vi "Delete.vi"(0 "image in":refnum<class "MSC Image.lvclass">, 5 "error in (no error)":errorcluster) -> (19 "error out":errorcluster)   [LabVIEW 2014, in "MSC Image.lvclass"]
doc: "Closes the image reference and frees occupied memory.\nUse this function for each initialized image to prevent memory leaks."
uses:
  MSC Image.lvclass
  MSC Image.lvclass/MSC Image.ctl
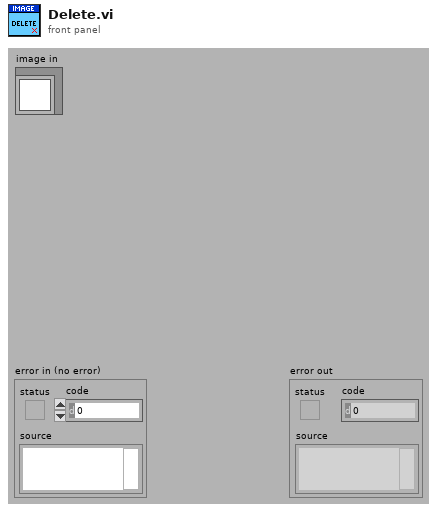
[diagram p1: front panel]
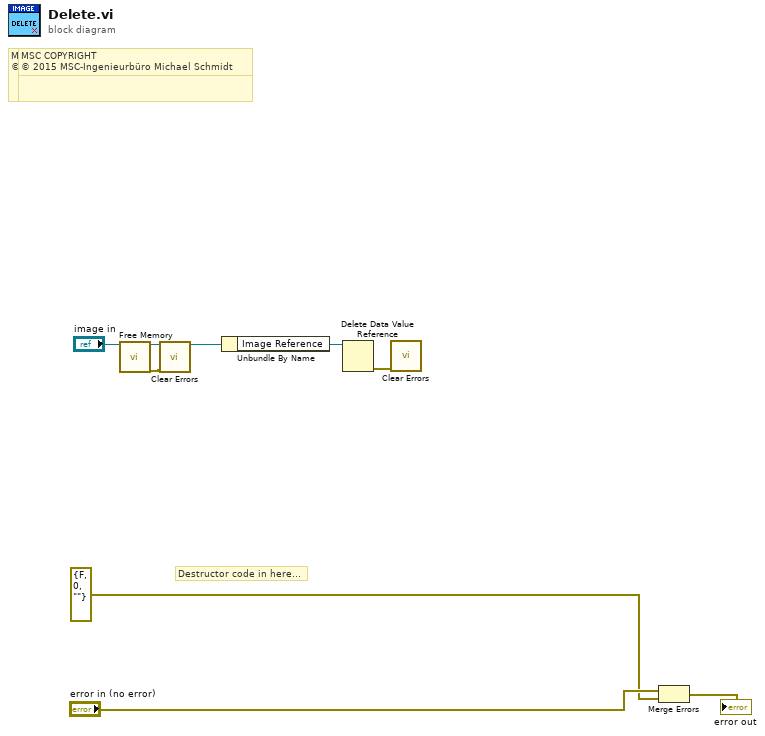
[diagram p0: block diagram]
diagram:
  # "MSC COPYRIGHT\n© 2016 MSC-Ingenieurbüro Michael Schmidt"
  # "MSC COPYRIGHT\n© 2016 MSC-Ingenieurbüro Michael Schmidt"
  # "MSC COPYRIGHT\n© 2015 MSC-Ingenieurbüro Michael Schmidt"
  # "MSC COPYRIGHT\n© 2015 MSC-Ingenieurbüro Michael Schmidt"
  # "Destructor code in here..."
  n1 = call "Free Memory.vi"("image in"="image in") -> ("image out"=w2:refnum<class "MSC Image.lvclass">, "error out"=w1:errorcluster)  [unwired: 17 in]
  n2 = call <vilib>:"Clear Errors.vi"("error in (no error)"=w1) -> ()  [unwired: 5 in, 2 out]
  n3 = Unbundle By Name(w2) -> ("Image Reference"=w5:refnum<data-value>)
  n4 = Delete Data Value Reference(data value reference=w5) -> (error out=w4:errorcluster)  [unwired: 1 in, 1 out]
  n5 = call <vilib>:"Clear Errors.vi"("error in (no error)"=w4) -> ()  [unwired: 5 in, 2 out]
  n6 = Merge Errors("error in (no error)", errorcluster {"status"=FALSE, "code"=0, "source"=""} ("error in (no error)")) -> (→"error out":errorcluster)
